vi "Select Response.vi"(10 "Output":refnum<class "Response.lvclass">, 11 "Input":refnum<class "Response.lvclass">) -> (3 "Selected":refnum<class "Response.lvclass">)   [LabVIEW 2020, in "HTTP Server.lvlib" / "Server.lvclass"]
uses:
  Server.lvclass
  lv-http-util/HTTP Utils/Response/Response.lvclass
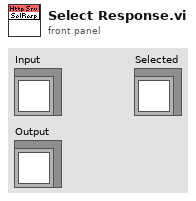
[diagram p1: front panel]
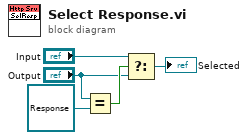
[diagram p0: block diagram]
diagram:
  n1 = Equal?(x="Output", y=refnum<class "Response.lvclass"> refnum) -> (x = y?=w3:bool)
  n2 = Select(t="Input", s=w3, f="Output") -> (s? t:f=→"Selected":refnum<class "Response.lvclass">)
